vi "CommFGV.vi"(7 "?":T1=enum."GetEventRefs", 8 "Error In":errorcluster) -> (0 "error out":errorcluster)   [LabVIEW 2017]
uses:
  TypeDefs/DataCluster.ctl
  MainFrameLib.lvlib
  TypeDefs/Command_Enum.ctl
  TypeDefs/FGV_Enum.ctl
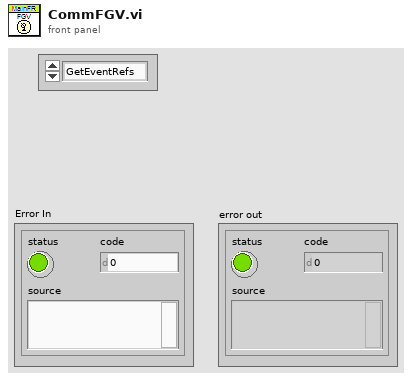
[diagram p1: front panel]
types:
  T1 = typedef "MainFrameLib.lvlib/FGV_Enum.ctl" = enum16{"Close", "GetEventRefs", "Set"}
  T2 = typedef "MainFrameLib.lvlib/DataCluster.ctl" = cluster{"Command":T3, "Data":variant}
  T3 = typedef "MainFrameLib.lvlib/Command_Enum.ctl" = enum16{"GetSRNotes", "DisplayAEStats", "InWork&Neglected", "RemapAENames", "ClearFolder", "UpdateReportsList", "ExcelReports", "TeamStats", "LoadReport", "WaitOnReport", "RequestReport", "Error", "Idle", "Initialize", "ScreenPop", "ClipboardCopy", "Shutdown"}
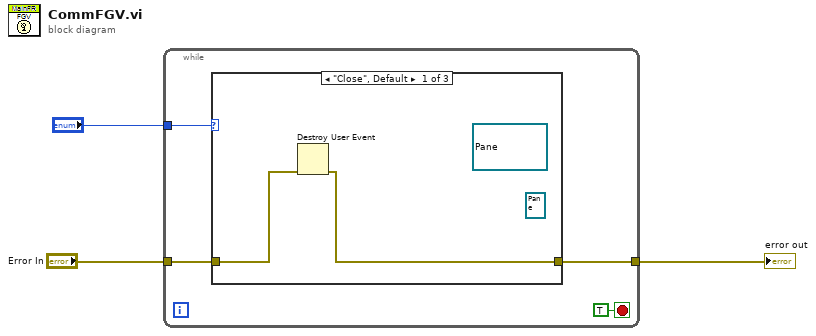
[diagram p0: block diagram]
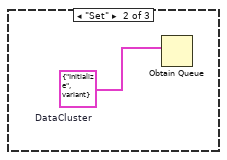
[diagram p2: hidden frame]
diagram:
  n1 = while {
    tunnel: "?" -> [w6]
    tunnel: "Error In" -> [w5]
    tunnel: [w4] -> w1
    stop <- TRUE stop-if-true
    n2 = case shown="\"Close\", Default" w6 {
      tunnel: w5 -> [w9 _ w11]
      tunnel: [w8 _ w11] -> w4
      frame "Close", Default {
        (unwired) refnum<event-registration> refnum ("Event Registration Refnum")
        (unwired) refnum<user-event> refnum ("DataEvent")
        n3 = Destroy User Event(error in=w9) -> (error out=w8:errorcluster)  [unwired: 1 in]
      }
      frame "Set" {
        w10 = T2 {"Command"=enum."Initialize", "Data"=variant}  # DataCluster
        n4 = Obtain Queue(element data type=w10) -> ()  [unwired: 4 in, 3 out]
      }
      frame "GetEventRefs" {
      }
    }
  }
  "error out" <- w1
